vi "Conversion Lookup Table Get Conversion Parameter.vi"(8 "error in (no error)":errorcluster, 10 "ID":u32, 11 "DVR":refnum<data-value>) -> (0 "error out":errorcluster {"code" min=0 max=0}, 1 "Found?":bool, 2 "Parameters":T1, 3 "DVR out":refnum<data-value>)   [LabVIEW 2013, in "J1939 Addon Engine.lvlib"]
uses:
  J1939 Addon Engine.lvlib
  Types/Conversion Lookup Table Parameters Cluster.ctl
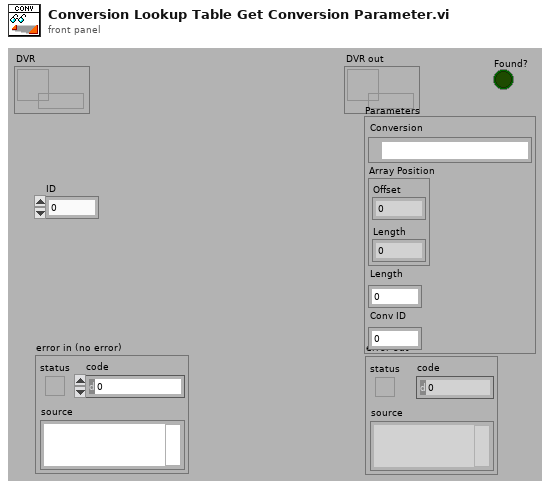
[diagram p1: front panel]
types:
  T1 = typedef "J1939 Addon Engine.lvlib/Conversion Lookup Table Parameters Cluster.ctl" = cluster{"Conversion":refnum<k21>, "Array Position":cluster{"Offset":u32, "Length":u32}, "Length":u32, "Conv ID":u32}
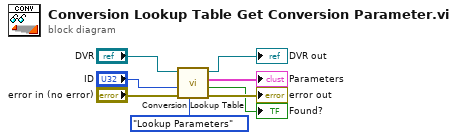
[diagram p0: block diagram]
diagram:
  n1 = call "Conversion Lookup Table.vi"("command"=enum16{"Set All", "Lookup Parameters"}."Lookup Parameters", "error in (no error)"="error in (no error)", "ID"="ID", "DVR"="DVR") -> ("error out"=→"error out":errorcluster, "Found?"=→"Found?":bool, "Parameters"=→"Parameters":T1, "DVR out"=→"DVR out":refnum<data-value>)  [unwired: 4 in]
